vi "hall.vi"() -> ()   [LabVIEW 2020]
uses:
  <vilib>/Instr/_visa.llb/VISA Configure Serial Port (Instr).vi
panel:
  in  "delay":u32=10
  out "Waveform Chart":dbl(graph)
  out "Data":string
  in  "stop":bool
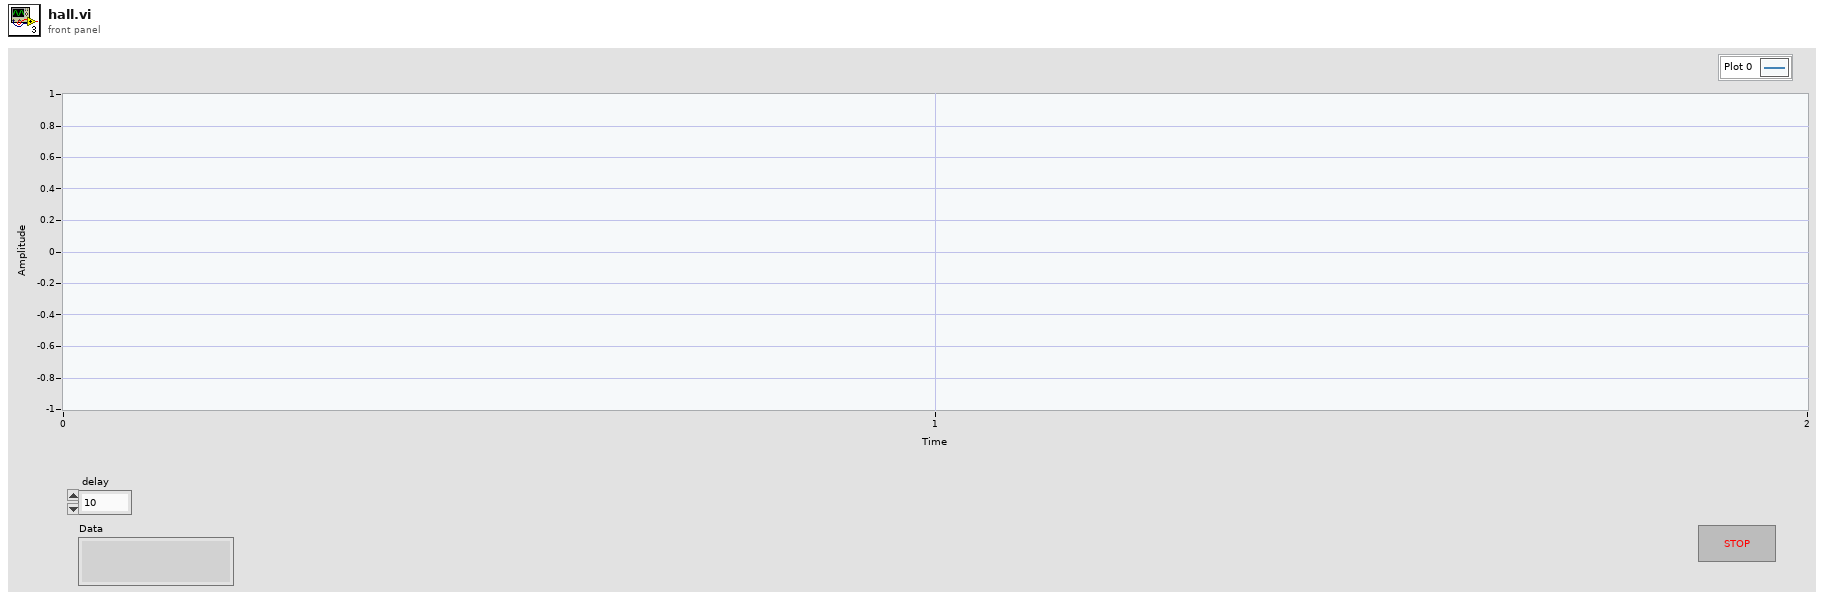
[diagram p1: front panel]
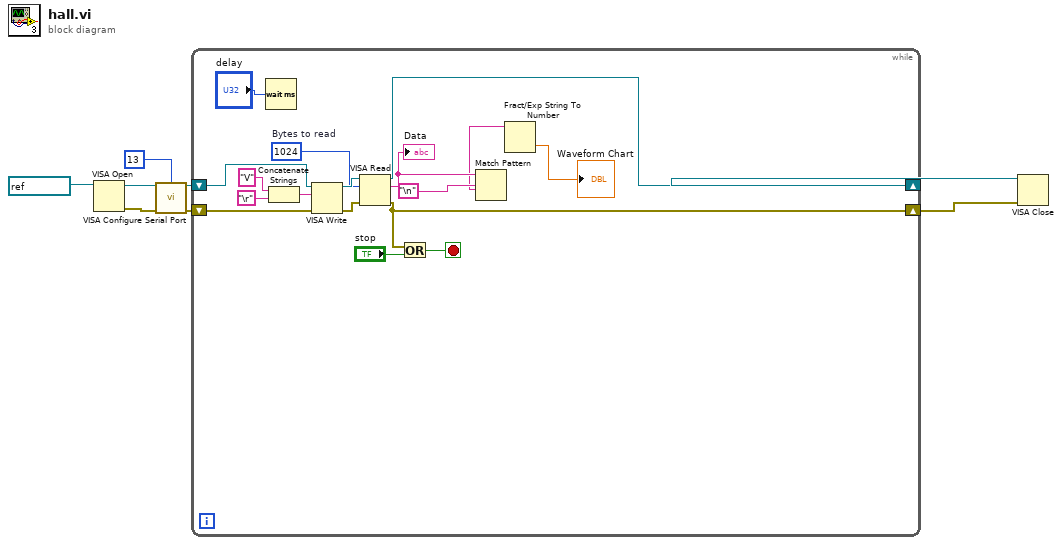
[diagram p0: block diagram]
diagram:
  n1 = VISA Open(VISA resource name=refnum<visa-resource-name> "COM5") -> (VISA resource name=w8:refnum<visa-resource-name>, error out=w7:errorcluster)  [unwired: 4 in]
  n2 = call-poly "VISA Configure Serial Port"("VISA resource name"=w8, "termination char\n(0xA = '\\n' = LF)"=u8 13 ("termination char\n(0xA = '\\n' = LF)"), "error in (no error)"=w7) -> ("VISA resource name out"=w6:refnum<visa-resource-name>, "error out"=w5:errorcluster)  [unwired: 11 in]
  n3 = while {
    shift-right: [w21] -> w4
    shift-left: w6 -> [w25]
    shift-right: [w16] -> w3
    shift-left: w5 -> [w24]
    stop <- w15 stop-if-true
    w20 = u32 1024  # Bytes to read
    n4 = Wait (ms)(milliseconds to wait="delay") -> ()  [unwired: 1 out]
    n5 = Concatenate Strings("V" ("write buffer"), "\r") -> (w18:string)
    n6 = VISA Write(VISA resource name=w25, write buffer=w18, error in (no error)=w24) -> (VISA resource name out=w23:refnum<visa-resource-name>, error out=w22:errorcluster)  [unwired: 1 out]
    n7 = VISA Read(VISA resource name=w23, byte count=w20, error in (no error)=w22) -> (VISA resource name out=w21:refnum<visa-resource-name>, read buffer=w12:string, error out=w16:errorcluster)  [unwired: 1 out]
    "Data" <- w12
    n8 = Or(x=w16, y="stop") -> (x .or. y?=w15:bool)
    n9 = Match Pattern(string=w12, regular expression="\n") -> (after substring=w11:string)  [unwired: 1 in, 3 out]
    n10 = Fract/Exp String To Number(string=w11) -> (number=→"Waveform Chart":dbl)  [unwired: 3 in, 1 out]
  }
  n11 = VISA Close(VISA resource name=w4, error in (no error)=w3) -> ()  [unwired: 1 out]
